vi "Save Intensity Dep Data.vi"(0 "Experiment Indicator":string, 1 "No. of Suns":dbl, 3 "Scan direction":i32, 4 "Data Array":dbl[][](array[numeric]), 6 "Username":string, 7 "Stabilisation time (ms)":dbl, 8 "Cell details cluster":T1={"Cell Position"=16, "Cell Label"="", "Pixel to measure"=0, "Area (cm^2)"=0.126, "Variable"="", "Variable value"="", "Scan settings in queue"=0, "Light or dark"="", "Measurement Type"=""} {"Pixel to measure" items=["All", "1", "2", "3", "4", "5", "6", "7", "8"]}, 10 "Measurement Delay (ms)":dbl=1.0, 11 "Stabilisation level \n(A or V depending on mode)":dbl=-1.4, 13 "Stabilisation Data":dbl[][](array[numeric])) -> (14 "Master Log":string[][](table), 15 "File path for master log":path, 17 "File path for JV data":path, 18 "File path for JV image":path)   [LabVIEW 2011]
uses:
  <vilib>/Utility/file.llb/Write To Spreadsheet File (string).vi
  <vilib>/Utility/file.llb/Read From Spreadsheet File (string).vi
  <vilib>/Analysis/NI_AALPro.lvlib
panel:
  in  "Scan rate (V/s)":dbl
  out "Vmp":dbl
  out "PCE":dbl
  out "FF":dbl
  out "Voc":dbl
  out "Jsc":dbl
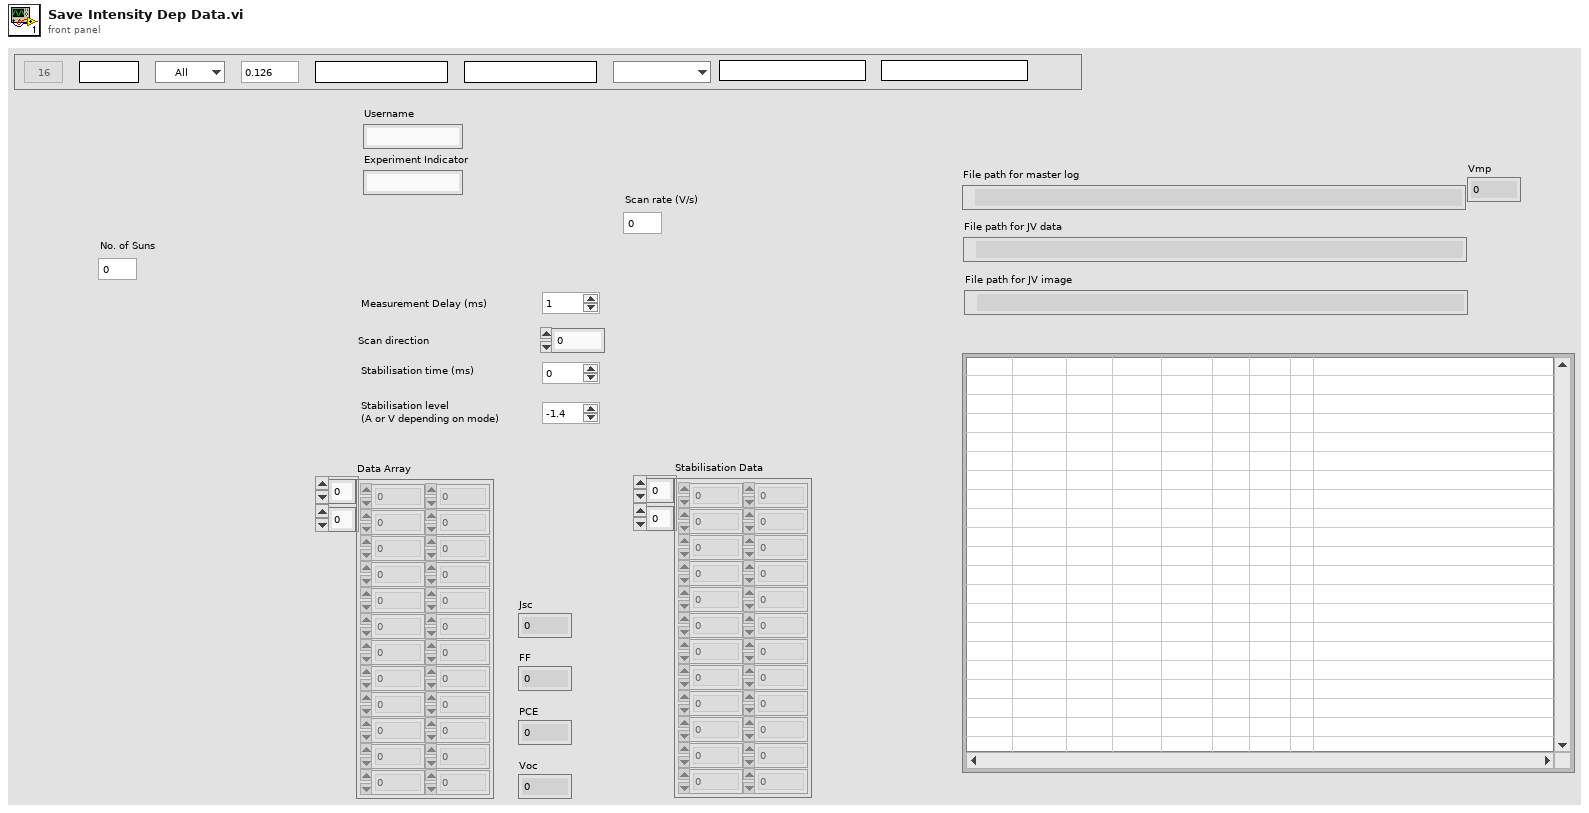
[diagram p1: front panel]
types:
  T1 = cluster{"Cell Position":i32, "Cell Label":string, "Pixel to measure":u16, "Area (cm^2)":dbl, "Variable":string, "Variable value":string, "Scan settings in queue":u16, "Light or dark":string, "Measurement Type":string}
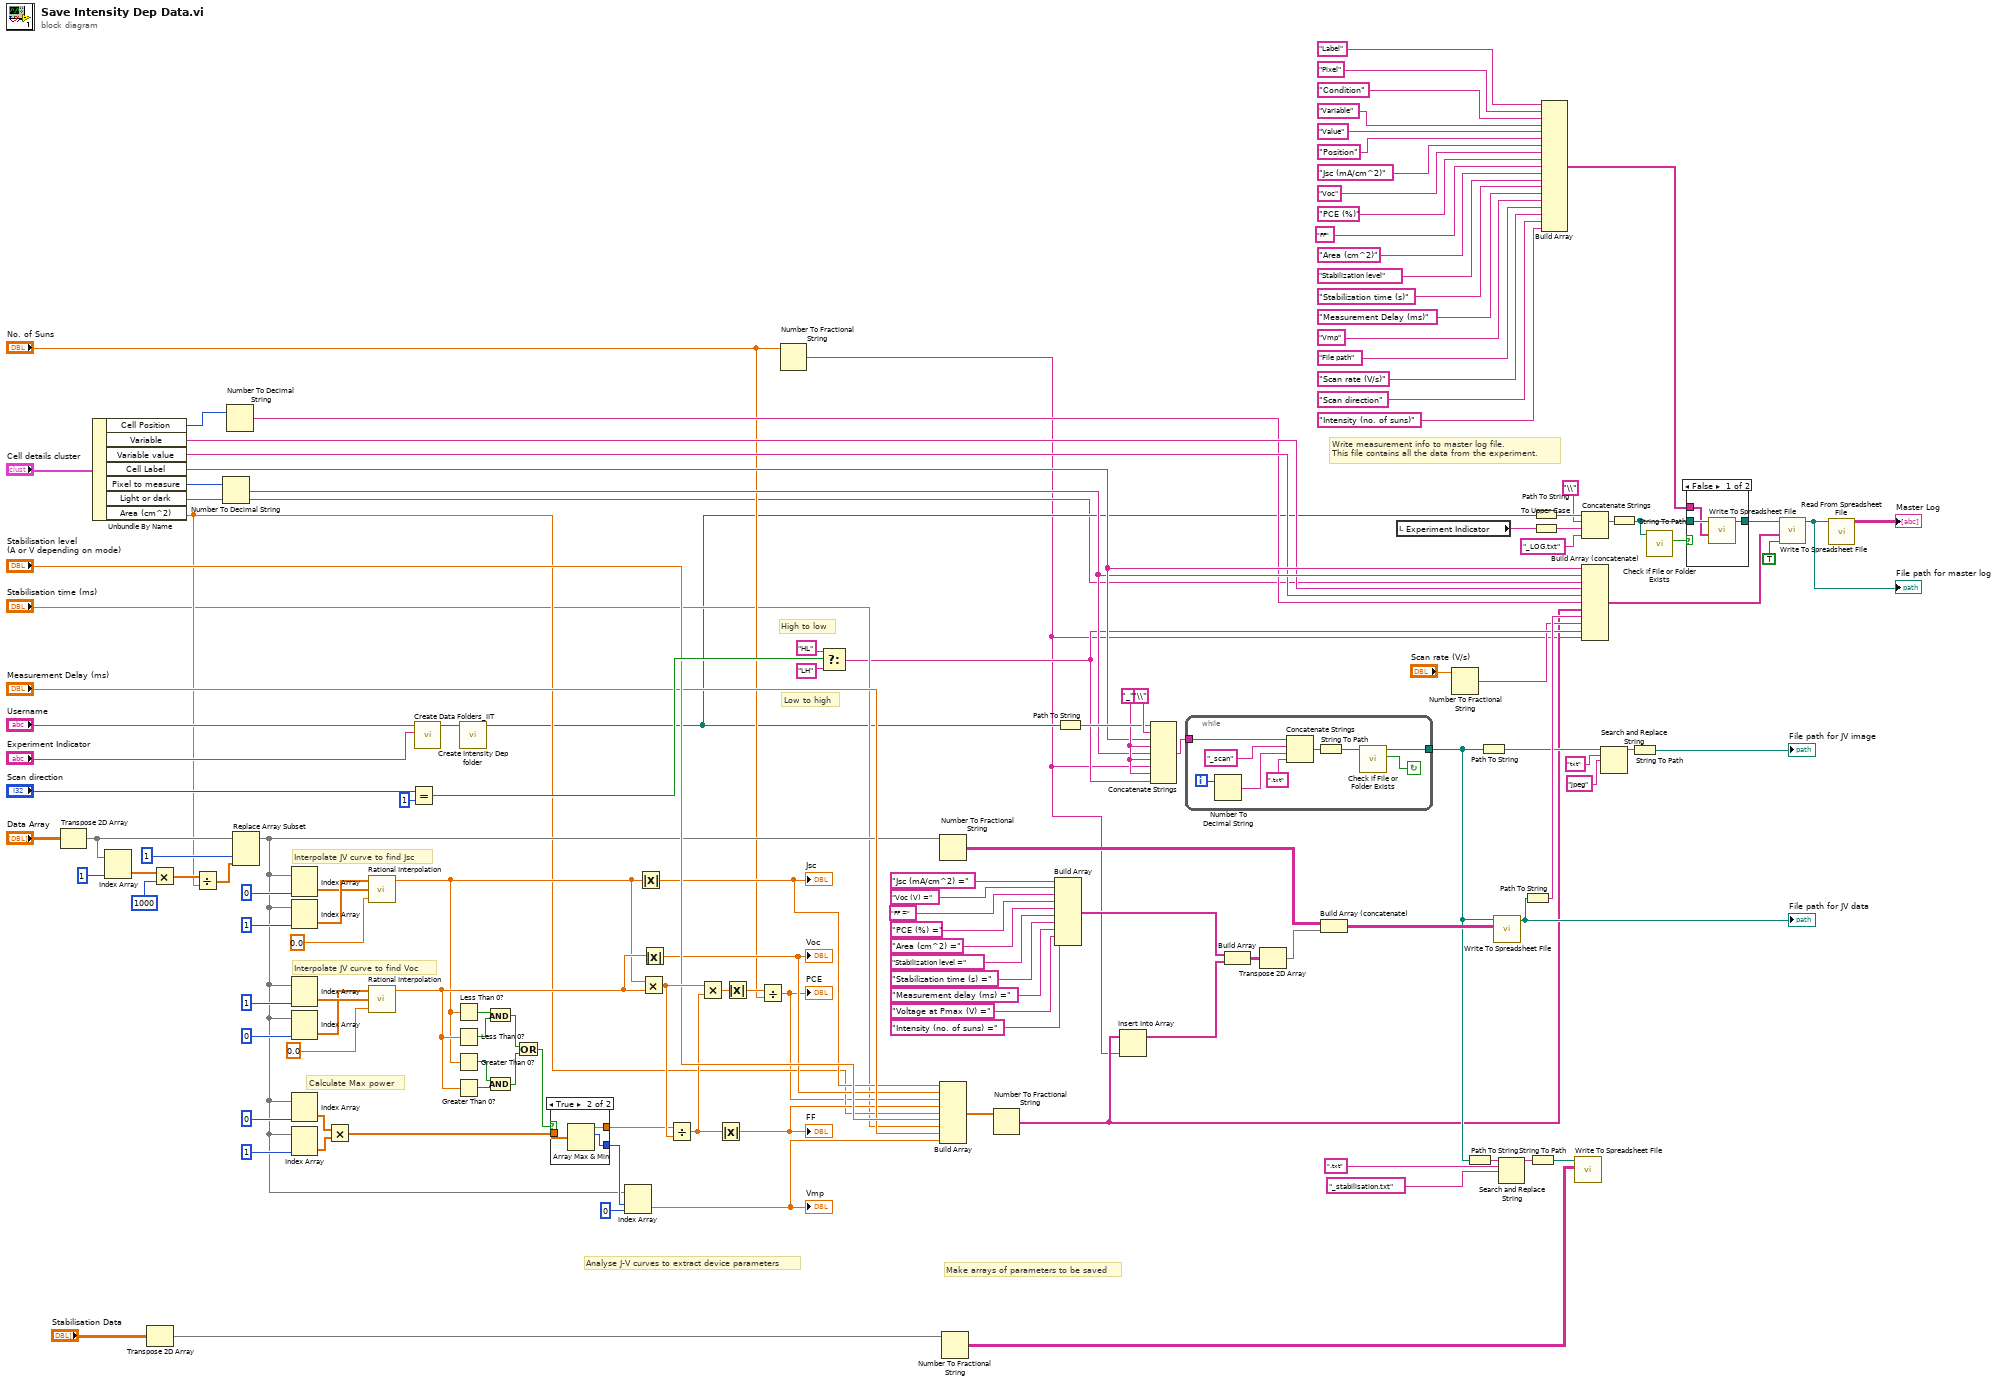
[diagram p0: block diagram]
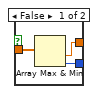
[diagram p3: hidden frame]
diagram:
  w61 = "_"
  # "Make arrays of parameters to be saved"
  # "Calculate Max power"
  # "Interpolate JV curve to find Voc"
  # "Interpolate JV curve to find Jsc"
  # "Analyse J-V curves to extract device parameters"
  # "Write measurement info to master log file.\nThis file contains all the data from the experiment."
  # "Low to high"
  # "High to low"
  n1 = Transpose 2D Array(2D array="Data Array") -> (transposed array=w69:dbl[][])
  n2 = Unbundle By Name("Cell details cluster") -> ("Cell Position"=w43:i32, "Variable"=w40:string, "Variable value"=w39:string, "Cell Label"=w42:string, "Pixel to measure"=w44:u16, "Light or dark"=w8:string, "Area (cm^2)"=w45:dbl)
  n3 = Index Array(array=w69, index (col)=1) -> (element=w67:dbl[])  [unwired: 1 in]
  n4 = Transpose 2D Array(2D array="Stabilisation Data") -> (transposed array=w52:dbl[][])
  n5 = Multiply(x=w67, y=1000) -> (x*y=w64:dbl[])
  n6 = Divide(x=w64, y=w45) -> (x/y=w63:dbl[])
  n7 = Number To Decimal String(number=w44) -> (decimal integer string=w41:string)  [unwired: 1 in]
  n8 = Number To Decimal String(number=w43) -> (decimal integer string=w38:string)  [unwired: 1 in]
  n9 = Replace Array Subset(array=w69, new element=w63, index (col)=1) -> (w49:dbl[][])  [unwired: 1 in]
  n10 = Index Array(array=w49, index (col)=0) -> (element=w132:dbl[])  [unwired: 1 in]
  n11 = Index Array(array=w49, index (col)=1) -> (element=w133:dbl[])  [unwired: 1 in]
  n12 = Index Array(array=w49, index (col)=1) -> (element=w131:dbl[])  [unwired: 1 in]
  n13 = Index Array(array=w49, index (col)=0) -> (element=w129:dbl[])  [unwired: 1 in]
  n14 = Index Array(array=w49, index (col)=0) -> (element=w137:dbl[])  [unwired: 1 in]
  n15 = Index Array(array=w49, index (col)=1) -> (element=w136:dbl[])  [unwired: 1 in]
  n16 = Multiply(x=w137, y=w136) -> (x*y=w130:dbl[])
  n17 = call <vilib>:"Rational Interpolation.vi"("x value"=0.0, "X"=w132, "Y"=w133) -> ("interpolation value"=w65:dbl)  [unwired: 2 out]
  n18 = call <vilib>:"Rational Interpolation.vi"("x value"=0.0, "X"=w131, "Y"=w129) -> ("interpolation value"=w75:dbl)  [unwired: 2 out]
  n19 = Equal?(x="Scan direction", y=1) -> (x = y?=w96:bool)
  n20 = call "Create Data Folders_IIT.vi"("Experiment Indicator"="Experiment Indicator", "username"="Username") -> ("Data Output Folder"=w16:path)  [unwired: 9 in]
  n21 = Less Than 0?(x=w65) -> (x < 0?=w81:bool)
  n22 = Less Than 0?(x=w75) -> (x < 0?=w78:bool)
  n23 = Greater Than 0?(x=w65) -> (x > 0?=w79:bool)
  n24 = Greater Than 0?(x=w75) -> (x > 0?=w80:bool)
  n25 = call "Create Intensity Dep folder.vi"("Data Folder In"=w16) -> ("Data Output Folder"=w15:path)  [unwired: 10 in]
  n26 = And(x=w81, y=w78) -> (x .and. y?=w83:bool)
  n27 = And(x=w79, y=w80) -> (x .and. y?=w82:bool)
  n28 = Or(x=w83, y=w82) -> (x .or. y?=w77:bool)
  n29 = case shown="True" w77 {
    tunnel: [w145 w149] -> w62
    tunnel: w130 -> [w146 w148]
    tunnel: [w144 w147] -> w50
    frame False {
      n30 = Array Max & Min(array=w146) -> (min value=w145:dbl, min index (indices)=w144:i32)  [unwired: 2 out]
    }
    frame True {
      n31 = Array Max & Min(array=w148) -> (max value=w149:dbl, max index (indices)=w147:i32)  [unwired: 2 out]
    }
  }
  n32 = Index Array(array=w49, index (row)=w50, index (col)=0) -> (element=w47:dbl)
  "Vmp" <- w47
  n33 = Absolute Value(x=w65) -> (abs(x)=w76:dbl)
  "Jsc" <- w76
  n34 = Multiply(x=w65, y=w75) -> (x*y=w128:dbl)
  n35 = Absolute Value(x=w75) -> (abs(x)=w74:dbl)
  "Voc" <- w74
  n36 = Divide(x=w62, y=w128) -> (x/y=w72:dbl)
  n37 = Multiply(x=w128, y=w72) -> (x*y=w73:dbl)
  n38 = Absolute Value(x=w72) -> (abs(x)=w71:dbl)
  "FF" <- w71
  n39 = Absolute Value(x=w73) -> (abs(x)=w19:dbl)
  n40 = Divide(x=w19, y="No. of Suns") -> (x/y=w20:dbl)
  "PCE" <- w20
  n41 = Number To Fractional String(number="No. of Suns") -> (F-format string=w1:string)  [unwired: 3 in]
  n42 = Select(t="HL", s=w96, f="LH") -> (s? t:f=w7:string)
  n43 = Number To Fractional String(number=w49) -> (F-format string=w98:string[][])  [unwired: 3 in]
  n44 = Build Array(w76, w74, w20, w71, w45, "Stabilisation level \n(A or V depending on mode)", "Stabilisation time (ms)", "Measurement Delay (ms)", w47) -> (w123:dbl[])
  n45 = Number To Fractional String(number=w52) -> (F-format string=w53:string[][])  [unwired: 3 in]
  n46 = Number To Fractional String(number=w123) -> (F-format string=w3:string[])  [unwired: 3 in]
  n47 = Build Array("Jsc (mA/cm^2) =", "Voc (V) =", "FF =", "PCE (%) =", "Area (cm^2) =", "Stabilization level =", "Stabilization time (s) =", "Measurement delay (ms) =", "Voltage at Pmax (V) =", "Intensity (no. of suns) =") -> (w122:string[])
  n48 = Path To String(path=w15) -> (string=w107:string)
  n49 = Insert Into Array(array=w3, new element=w1) -> (w2:string[])  [unwired: 1 in]
  n50 = Concatenate Strings(w107, "\\", w42, w61, w41, w61, w1, w61, w7) -> (w88:string)
  n51 = while {
    tunnel: w88 -> [w158]
    tunnel: [w150] -> w59
    i -> [w156]
    stop <- w151 continue-if-true
    n52 = Number To Decimal String(number=w156) -> (decimal integer string=w155:string)  [unwired: 1 in]
    n53 = Concatenate Strings(w158, "_scan", w155, ".txt") -> (w152:string)
    n54 = String To Path(string=w152) -> (path=w153:path)
    n55 = call <vilib>:"Check if File or Folder Exists.vi"("path"=w153) -> ("file or folder exists?"=w151:bool, "dup path"=w150:path)  [unwired: 8 in, 1 out]
  }
  n56 = Build Array(w122, w2) -> (w118:string[][])
  n57 = Transpose 2D Array(2D array=w118) -> (transposed array=w117:string[][])
  n58 = Build Array (concatenate)(w98, w117) -> (w121:string[][])
  n59 = local read "Experiment Indicator"() -> (w84:string)
  n60 = Number To Fractional String(number="Scan rate (V/s)") -> (F-format string=w5:string)  [unwired: 3 in]
  n61 = Path To String(path=w59) -> (string=w58:string)
  n62 = Path To String(path=w59) -> (string=w87:string)
  n63 = call-poly <vilib>:"Write To Spreadsheet File.vi"("2D data"=w121, "file path (dialog if empty)"=w59) -> ("new file path (Not A Path if cancelled)"=w94:path)  [unwired: 6 in]
  "File path for JV data" <- w94
  n64 = Search and Replace String(input string=w58, search string=".txt", replace string="_stabilisation.txt") -> (result string=w55:string)  [unwired: 5 in, 3 out]
  n65 = Path To String(path=w94) -> (string=w89:string)
  n66 = String To Path(string=w55) -> (path=w54:path)
  n67 = Path To String(path=w15) -> (string=w113:string)
  n68 = To Upper Case(1:w84) -> (0:w85:string)
  n69 = Build Array("Label", "Pixel", "Condition", "Variable", "Value", "Position", "Jsc (mA/cm^2)", "Voc", "PCE (%)", "FF", "Area (cm^2)", "Stabilization level", "Stabilization time (s)", "Measurement Delay (ms)", "Vmp", "File path", "Scan rate (V/s)", "Scan direction", "Intensity (no. of suns)") -> (w21:string[])
  n70 = call-poly <vilib>:"Write To Spreadsheet File.vi"("2D data"=w53, "file path (dialog if empty)"=w54) -> ()  [unwired: 6 in, 1 out]
  n71 = Concatenate Strings(w113, "\\", w85, "_LOG.txt") -> (w111:string)
  n72 = Build Array (concatenate)(w42, w41, w8, w40, w39, w38, w3, w89, w5, w7, w1) -> (w110:string[])
  n73 = Search and Replace String(input string=w87, search string="txt", replace string="jpeg") -> (result string=w106:string)  [unwired: 5 in, 3 out]
  n74 = String To Path(string=w111) -> (path=w23:path)
  n75 = String To Path(string=w106) -> (path=→"File path for JV image":path)
  n76 = call <vilib>:"Check if File or Folder Exists.vi"("path"=w23) -> ("file or folder exists?"=w24:bool)  [unwired: 8 in, 2 out]
  n77 = case shown="False" w24 {
    tunnel: w23 -> [w161 w162]
    tunnel: [w160 w162] -> w22
    tunnel: w21 -> [w159 _]
    frame False {
      n78 = call-poly <vilib>:"Write To Spreadsheet File.vi"("1D data"=w159, "file path (dialog if empty)"=w161) -> ("new file path (Not A Path if cancelled)"=w160:path)  [unwired: 6 in]
    }
    frame True {
    }
  }
  n79 = call-poly <vilib>:"Write To Spreadsheet File.vi"("append to file? (new file:F)"=TRUE, "1D data"=w110, "file path (dialog if empty)"=w22) -> ("new file path (Not A Path if cancelled)"=w101:path)  [unwired: 5 in]
  "File path for master log" <- w101
  n80 = call-poly <vilib>:"Read From Spreadsheet File.vi"("file path (dialog if empty)"=w101) -> ("all rows"=→"Master Log":string[][])  [unwired: 6 in, 4 out]
